vi "set_commands.vi"(8 "error in (no error)":errorcluster, 10 "commands":refnum<class "command_generic.lvclass">[](array[class]), 11 "Protocol_Generic in":refnum<class "Protocol_Generic.lvclass">) -> (0 "error out":errorcluster, 3 "Protocol_Generic out":refnum<class "Protocol_Generic.lvclass">)   [LabVIEW 2015, in "Protocol_Generic.lvclass"]
uses:
  Protocol_Generic.lvclass
  command/command_generic.lvclass
  Protocol_Generic.lvclass/Protocol_Generic.ctl
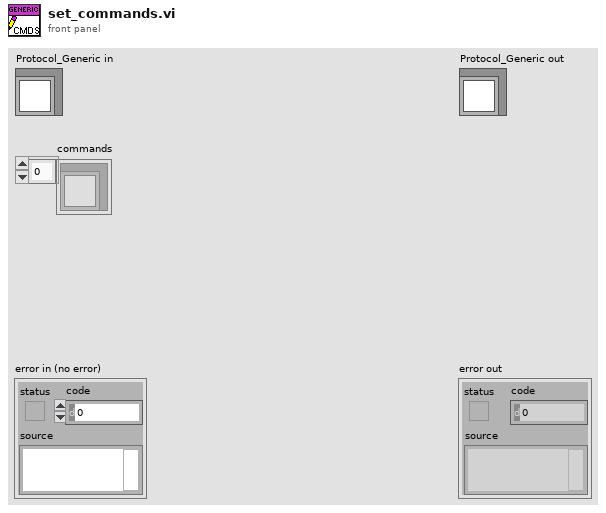
[diagram p1: front panel]
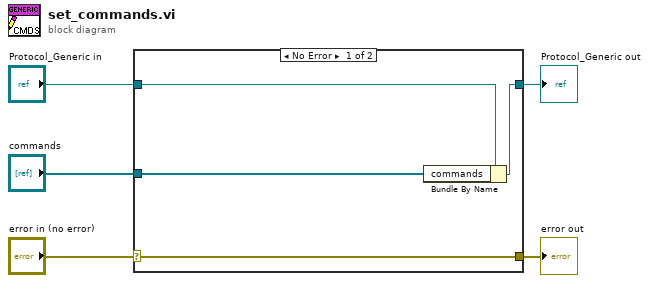
[diagram p0: block diagram]
diagram:
  n1 = case shown="No Error" "error in (no error)" {
    selector: "error in (no error)" -> [w9 w10]
    tunnel: [w9 w10] -> w4
    tunnel: [w7 w11] -> w2
    tunnel: "Protocol_Generic in" -> [w8 w11]
    tunnel: "commands" -> [w6 _]
    frame No Error {
      n2 = Bundle By Name(cluster=w8, "commands"=w6) -> (w7:refnum<class "Protocol_Generic.lvclass">)
    }
    frame Error {
    }
  }
  "error out" <- w4
  "Protocol_Generic out" <- w2
